vi "GlobalData.vi"() -> ()   [LabVIEW 2017]
uses:
  Controls/ShiftRegisterCluster.ctl
panel:
  in  "Data Cluster":T1
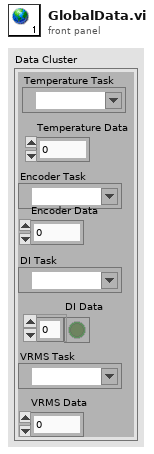
[diagram p1: front panel]
types:
  T1 = typedef "ShiftRegisterCluster.ctl" = cluster{"Temperature Task":refnum<k21>, "Temperature Data":dbl, "Encoder Task":refnum<k21>, "Encoder Data":dbl, "DI Task":refnum<k21>, "DI Data":bool[], "VRMS Task":refnum<k21>, "VRMS Data":dbl}
diagram:
